vi "源配置.vi"(7 "Item":string, 8 "error in (no error)":errorcluster caption="错误输入（无错误）", 10 "Arguments":string[](array[string]), 11 "多功能校准源接口输入":refnum<class "多功能校准源接口.lvclass">) -> (0 "error out":errorcluster caption="错误输出", 3 "多功能校准源接口输出":refnum<class "多功能校准源接口.lvclass">)   [LabVIEW 2020]
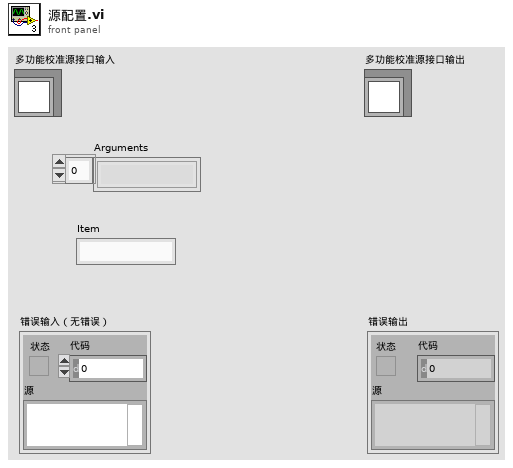
[diagram p1: front panel]
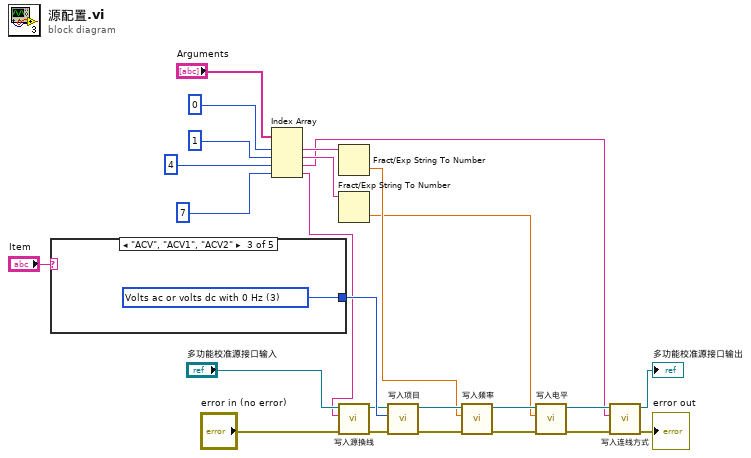
[diagram p0: block diagram]
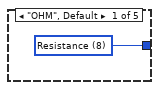
[diagram p2: hidden frame]
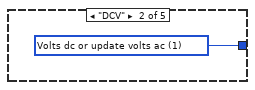
[diagram p3: hidden frame]
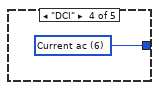
[diagram p4: hidden frame]
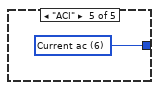
[diagram p5: hidden frame]
diagram:
  n1 = case shown="\"ACV\", \"ACV1\", \"ACV2\"" "Item" {
    tunnel: [w26 w27 w28 w29 w30] -> w12
    frame "OHM", Default {
      w26 = u32 8 items=["Amplitude", "Volts dc or update volts ac", "Volts ac dBm update", "Volts ac or volts dc with 0 Hz", "Volts ac in dBm", "Current dc or update current ac", "Current ac", "Update frequency", "Resistance", "Capacitance", "Temperature (Celsius)", "Temperature (Fahrenheit)", "Power dc or update power ac", "Power ac", "Dual volts dc or update dual ac", "Dual volts ac in volts", "Power ac in dBm update", "Power ac in dBm", "Dual volts ac in dBm update", "Dual volts ac in dBm"] ("项目")
    }
    frame "DCV" {
      w27 = u32 1 items=["Amplitude", "Volts dc or update volts ac", "Volts ac dBm update", "Volts ac or volts dc with 0 Hz", "Volts ac in dBm", "Current dc or update current ac", "Current ac", "Update frequency", "Resistance", "Capacitance", "Temperature (Celsius)", "Temperature (Fahrenheit)", "Power dc or update power ac", "Power ac", "Dual volts dc or update dual ac", "Dual volts ac in volts", "Power ac in dBm update", "Power ac in dBm", "Dual volts ac in dBm update", "Dual volts ac in dBm"] ("项目")
    }
    frame "ACV", "ACV1", "ACV2" {
      w28 = u32 3 items=["Amplitude", "Volts dc or update volts ac", "Volts ac dBm update", "Volts ac or volts dc with 0 Hz", "Volts ac in dBm", "Current dc or update current ac", "Current ac", "Update frequency", "Resistance", "Capacitance", "Temperature (Celsius)", "Temperature (Fahrenheit)", "Power dc or update power ac", "Power ac", "Dual volts dc or update dual ac", "Dual volts ac in volts", "Power ac in dBm update", "Power ac in dBm", "Dual volts ac in dBm update", "Dual volts ac in dBm"] ("项目")
    }
    frame "DCI" {
      w29 = u32 6 items=["Amplitude", "Volts dc or update volts ac", "Volts ac dBm update", "Volts ac or volts dc with 0 Hz", "Volts ac in dBm", "Current dc or update current ac", "Current ac", "Update frequency", "Resistance", "Capacitance", "Temperature (Celsius)", "Temperature (Fahrenheit)", "Power dc or update power ac", "Power ac", "Dual volts dc or update dual ac", "Dual volts ac in volts", "Power ac in dBm update", "Power ac in dBm", "Dual volts ac in dBm update", "Dual volts ac in dBm"] ("Output Value(s) (0 - Amplitude)")
    }
    frame "ACI" {
      w30 = u32 6 items=["Amplitude", "Volts dc or update volts ac", "Volts ac dBm update", "Volts ac or volts dc with 0 Hz", "Volts ac in dBm", "Current dc or update current ac", "Current ac", "Update frequency", "Resistance", "Capacitance", "Temperature (Celsius)", "Temperature (Fahrenheit)", "Power dc or update power ac", "Power ac", "Dual volts dc or update dual ac", "Dual volts ac in volts", "Power ac in dBm update", "Power ac in dBm", "Dual volts ac in dBm update", "Dual volts ac in dBm"] ("Output Value(s) (0 - Amplitude)")
    }
  }
  n2 = Index Array(array="Arguments", index #1=0 ("索引"), index #2=1 ("索引"), index #3=4 ("索引"), index #4=7 ("索引")) -> (element #1=w11:string, element #2=w21:string, element #3=w8:string, element #4=w2:string)
  n3 = Fract/Exp String To Number(string=w11) -> (number=w10:dbl)  [unwired: 3 in, 1 out]
  n4 = Fract/Exp String To Number(string=w21) -> (number=w9:dbl)  [unwired: 3 in, 1 out]
  n5 = call "写入源换线.vi"("error in (no error)"="error in (no error)", "源换线"=w2, "多功能校准源接口输入"="多功能校准源接口输入") -> ("error out"=w3:errorcluster, "多功能校准源接口输出"=w5:refnum<class "多功能校准源接口.lvclass">)  [unwired: 7 in]
  n6 = call "写入项目.vi"("error in (no error)"=w3, "项目"=w12, "多功能校准源接口输入"=w5) -> ("error out"=w19:errorcluster, "多功能校准源接口输出"=w18:refnum<class "多功能校准源接口.lvclass">)  [unwired: 7 in]
  n7 = call "写入频率.vi"("error in (no error)"=w19, "频率"=w10, "多功能校准源接口输入"=w18) -> ("error out"=w17:errorcluster, "多功能校准源接口输出"=w16:refnum<class "多功能校准源接口.lvclass">)  [unwired: 7 in]
  n8 = call "写入电平.vi"("error in (no error)"=w17, "电平"=w9, "多功能校准源接口输入"=w16) -> ("error out"=w15:errorcluster, "多功能校准源接口输出"=w14:refnum<class "多功能校准源接口.lvclass">)  [unwired: 7 in]
  n9 = call "写入连线方式.vi"("error in (no error)"=w15, "连线方式"=w8, "多功能校准源接口输入"=w14) -> ("error out"=→"error out":errorcluster, "多功能校准源接口输出"=→"多功能校准源接口输出":refnum<class "多功能校准源接口.lvclass">)  [unwired: 7 in]
